vi "Set DataCell (String).vi"(0 "DataTable in":refnum<class "DataTable.lvclass">, 1 "image path":path, 5 "row index":i32, 7 "col index":i32, 9 "String Data":string, 11 "error in (no error)":errorcluster) -> (4 "DataTable out":refnum<class "DataTable.lvclass">, 15 "error out":errorcluster)   [LabVIEW 2016, in "DataGrid.lvlib" / "DataTable.lvclass"]
doc: "This allows any number of rows to be added to the datatable. The data must match the columns defined for the grid."
uses:
  <userlib>/LabVIEWdotNetDataGrid/source/DataTable/DataTable.lvclass
  <userlib>/LabVIEWdotNetDataGrid/source/DataTable/DataTable.lvclass/DataTable.ctl
  System.Data
  <userlib>/LabVIEWdotNetDataGrid/source/GridColumn/GridColumn.lvclass/GridColumn.ctl
  <userlib>/LabVIEWdotNetDataGrid/source/GridColumn/Read datatype.vi
  <userlib>/LabVIEWdotNetDataGrid/source/GridColumn/GridColumn.lvclass
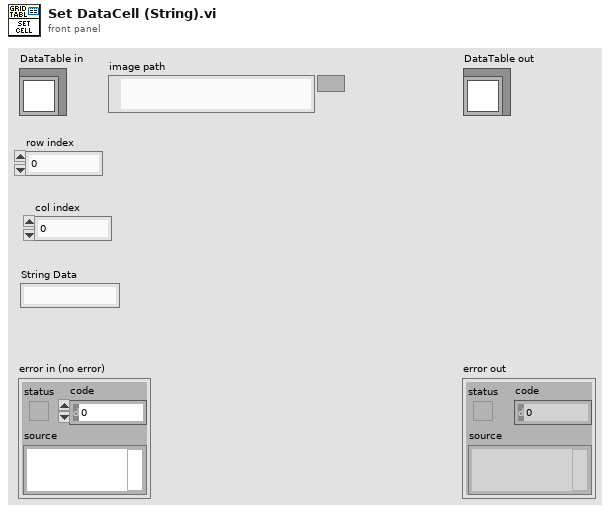
[diagram p1: front panel]
types:
  T1 = typedef "DataGrid.lvlib/GridColumn.lvclass/ColumnType.ctl" = enum16{"string", "image", "check", "numeric", "timestamp", "button", "combo", "link"}
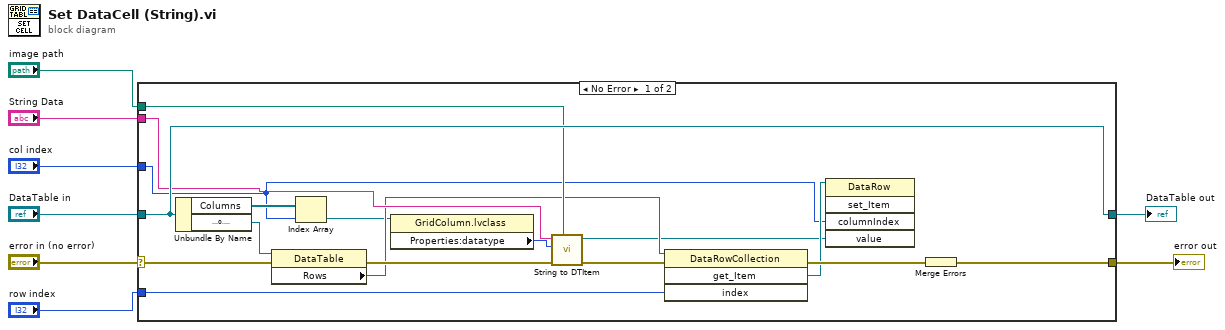
[diagram p0: block diagram]
diagram:
  n1 = case shown="No Error" "error in (no error)" {
    selector: "error in (no error)" -> [w22 w26]
    tunnel: [w23 w27] -> w6
    tunnel: "DataTable in" -> [w23 w27]
    tunnel: "String Data" -> [w21 _]
    tunnel: [w19 w26] -> w4
    tunnel: "image path" -> [w18 _]
    tunnel: "row index" -> [w13 _]
    tunnel: "col index" -> [w9 _]
    frame No Error {
      n2 = Unbundle By Name(w23) -> ("Columns"=w17:refnum<class "GridColumn.lvclass">[], "DataTable"=w20:refnum<k24>)
      n3 = property class="DataTable"(reference=w20, error in=w22) -> (error out=w25:errorcluster, "Rows"=w16:refnum<k24>)  [unwired: 1 out]
      n4 = Index Array(array=w17, index=w9) -> (element=w11:refnum<class "GridColumn.lvclass">)
      n5 = property class="GridColumn.lvclass"(reference=w11) -> ("Properties:datatype"=w12:T1)  [unwired: 1 in, 2 out]
      n6 = call <userlib>:"String to DTItem.vi"("image path"=w18, "error in (no error)"=w25, "datatype"=w12, "element"=w21) -> ("error out"=w15:errorcluster, "DTItem .NET Refnum out"=w10:refnum<k24>)  [unwired: 6 in]
      n7 = invoke class="DataRowCollection" method="get_Item"(reference=w16, error in=w15, "index"=w13) -> (error out=w24:errorcluster, "get_Item"=w14:refnum<k24>)  [unwired: 1 in, 2 out]
      n8 = invoke class="DataRow" method="set_Item"(reference=w14, "columnIndex"=w9, "value"=w10) -> ()  [unwired: 2 in, 5 out]
      n9 = Merge Errors(w24) -> (w19:errorcluster)
    }
    frame Error {
    }
  }
  "error out" <- w4
  "DataTable out" <- w6
